vi "Insert Static Panels.vi"(8 "error in (no error)":errorcluster, 11 "PanelArray in":refnum<class "PanelArray.lvclass">) -> (0 "error out":errorcluster, 3 "PanelArray out":refnum<class "PanelArray.lvclass">)   [LabVIEW 2018, in "OOPanel.lvlib" / "PanelArray.lvclass"]
uses:
  PanelArray.lvclass
  PanelArray.lvclass/PanelArray.ctl
  Panel/State.ctl
  Panel/Panel.lvclass
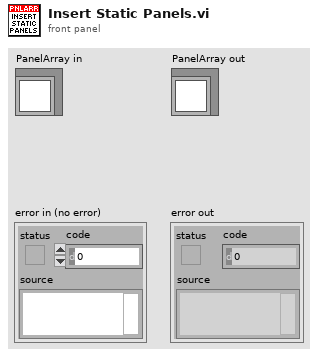
[diagram p1: front panel]
types:
  T1 = typedef "OOPanel.lvlib/PanelArray.lvclass/Ref Data.ctl" = cluster{"State":T2, "Refs":T3, "Events":T4, "Scrolling":T5, "Panels":T6}
  T2 = typedef "OOPanel.lvlib/PanelArray.lvclass/State.ctl" = cluster{"Defer Updates":bool, "Running":bool, "Dynamic Sizing":bool, "Borders":bool}
  T3 = typedef "OOPanel.lvlib/PanelArray.lvclass/Refs.ctl" = cluster{"SubPanels":refnum<vi>[], "Scrollbar":refnum<vi>, "Owning Panel":refnum<vi>}
  T4 = typedef "OOPanel.lvlib/PanelArray.lvclass/Events.ctl" = cluster{"Close":refnum<user-event>}
  T5 = typedef "OOPanel.lvlib/PanelArray.lvclass/Scrolling.ctl" = cluster{"Size":i32, "Max":i32, "Current":i32, "Top Index":i32, "Heights":i32[]}
  T6 = typedef "OOPanel.lvlib/PanelArray.lvclass/Panels.ctl" = cluster{"All":refnum<class "Panel.lvclass">[], "Visible":refnum<class "Panel.lvclass">[], "Blank":refnum<class "ArrayBlank.lvclass">}
  T7 = typedef "OOPanel.lvlib/Panel.lvclass/State.ctl" = enum16{"Idle", "Hidden", "Visible", "Subpanel"}
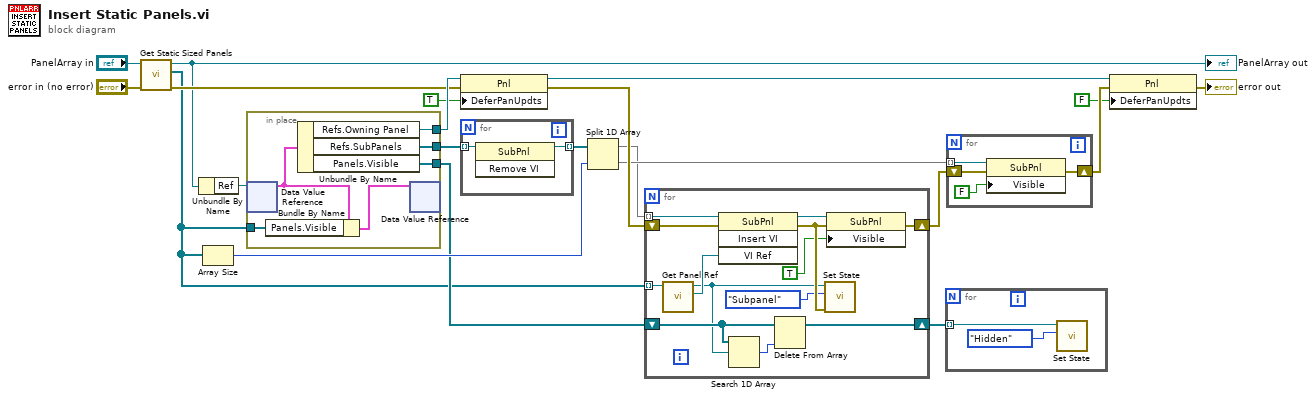
[diagram p0: block diagram]
diagram:
  n1 = call "Get Static Sized Panels.vi"("error in (no error)"="error in (no error)", "PanelArray in"="PanelArray in") -> ("error out"=w4:errorcluster, "Visible Panels"=w1:refnum<class "Panel.lvclass">[], "PanelArray out"=w2:refnum<class "PanelArray.lvclass">)  [unwired: 7 in]
  "PanelArray out" <- w2
  n2 = Unbundle By Name(w2) -> ("Ref"=w21:refnum<data-value>)
  n3 = Array Size(array=w1) -> (size(s)=w20:i32)
  n4 = in-place {
    in-place-border: [w27] -> w16
    in-place-border: w1 -> [w24]
    in-place-border: [w23] -> w19
    in-place-border: [w22] -> w12
    n5 = in-place-dvr #1(w21) -> (w26:T1)  [unwired: 1 out]
    n6 = Bundle By Name(cluster=w26, "Panels.Visible"=w24) -> (w25:T1)
    n7 = Unbundle By Name(w26) -> ("Refs.Owning Panel"=w23:refnum<vi>, "Refs.SubPanels"=w27:refnum<vi>[], "Panels.Visible"=w22:refnum<class "Panel.lvclass">[])
    n8 = in-place-dvr #1(w25) -> ()  [unwired: 2 out]
  }
  n9 = property class="Pnl"(reference=w19, error in=w4, "DeferPanUpdts"=TRUE ("Defer Panel Updates")) -> (reference out=w6:refnum<vi>, error out=w17:errorcluster)
  n10 = for {
    tunnel: w16 -> [w29] mode=indexing
    tunnel: [w28] -> w15 mode=indexing
    n11 = invoke class="SubPnl" method="Remove VI"(reference=w29) -> (reference out=w28:refnum<vi>)  [unwired: 2 in, 2 out]
  }
  n12 = Split 1D Array(array=w15, index=w20) -> (first subarray=w10:refnum<vi>[], second subarray=w14:refnum<vi>[])
  n13 = for {
    tunnel: w1 -> [w41] mode=indexing
    tunnel: w10 -> [w40] mode=indexing
    shift-right: [w37] -> w13
    shift-left: w17 -> [w39]
    shift-right: [w34] -> w11
    shift-left: w12 -> [w36]
    n14 = call "Get Panel Ref.vi"("Panel in"=w41) -> ("Panel Ref"=w32:refnum<vi>, "Panel out"=w30:refnum<class "Panel.lvclass">)  [unwired: 8 in, 1 out]
    n15 = invoke class="SubPnl" method="Insert VI"(reference=w40, error in=w39, "VI Ref"=w32) -> (reference out=w38:refnum<vi>, error out=w42:errorcluster)  [unwired: 1 in, 2 out]
    n16 = Search 1D Array(1D array=w36, element=w30) -> (index of element=w35:i32)  [unwired: 1 in]
    n17 = Delete From Array(array=w36, index=w35) -> (array with subset deleted=w34:refnum<class "Panel.lvclass">[])  [unwired: 1 in, 1 out]
    n18 = call "Set State.vi"("error in (no error)"=w42, "State"=State."Subpanel", "Panel in"=w30) -> ()  [unwired: 7 in, 2 out]
    n19 = property class="SubPnl"(reference=w38, error in=w42, "Visible"=TRUE) -> (error out=w37:errorcluster)  [unwired: 1 out]
  }
  n20 = for {
    tunnel: w11 -> [w43] mode=indexing
    n21 = call "Set State.vi"("State"=State."Hidden", "Panel in"=w43) -> ()  [unwired: 8 in, 2 out]
  }
  n22 = for {
    tunnel: w14 -> [w48] mode=indexing
    shift-right: [w45] -> w9
    shift-left: w13 -> [w47]
    n23 = property class="SubPnl"(reference=w48, error in=w47, "Visible"=FALSE) -> (error out=w45:errorcluster)  [unwired: 1 out]
  }
  n24 = property class="Pnl"(reference=w6, error in=w9, "DeferPanUpdts"=FALSE ("Defer Panel Updates")) -> (error out=→"error out":errorcluster)  [unwired: 1 out]
